vi "PH_Sound.ProcPeriodic.vi"(0 "i ref in":refnum<vi>, 3 "ms timeout (100)":i32=100, 5 "error in (no error)":errorcluster) -> (14 "i ref out":refnum<vi>, 17 "timed out":bool, 19 "error out":errorcluster)   [LabVIEW 2014, in "PH_Sound.lvlib"]
doc: "This method serves to periodically do things like reading values from the HW. Methods that should be executed periodically should be called from THIS methode. Add code here."
uses:
  PH_Sound.lvlib
  PH_Sound.3Oktaves.ctl
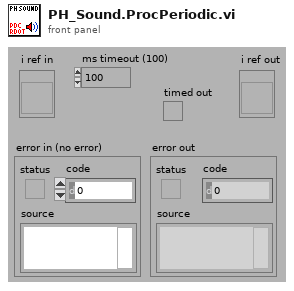
[diagram p1: front panel]
types:
  T1 = typedef "PH_Sound.lvlib/PH_Sound.i attribute.ctl" = cluster{"GUI Refs":cluster{"Exit":refnum<vi>, "Laserfreigabe":refnum<vi>, "PreAmp-Freigabe":refnum<vi>, "Countdown Running":refnum<vi>, "Emergency Off":refnum<vi>, "Device Error":refnum<vi>}, "Testalarm on":bool, "State":cluster{"Laser Class 4":bool, "PreAmp Running":bool, "Countdown Running":bool, "Emergency Off":bool}, "Starting Time":timestamp}
  T2 = typedef "PH_Sound.lvlib/PH_Sound.3Oktaves.ctl" = dbl
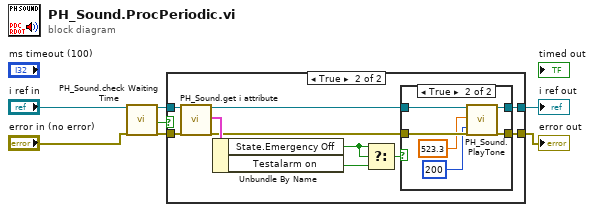
[diagram p0: block diagram]
diagram:
  n1 = call "PH_Sound.check Waiting Time.vi"("i ref in"="i ref in", "error in"="error in (no error)") -> ("i ref out"=w2:refnum<vi>, "Waiting Time over?"=w1:bool, "error out"=w4:errorcluster)  [unwired: 15 in]
  n2 = case shown="True" w1 {
    tunnel: [w9 w10] -> w7
    tunnel: [w8 w17] -> w6
    tunnel: w4 -> [w8 w12]
    tunnel: w2 -> [w9 w13]
    frame False {
    }
    frame True {
      n3 = call "PH_Sound.get i attribute.vi"("i ref in"=w13, "error in (no error)"=w12) -> ("i ref out"=w11:refnum<vi>, "i attribute"=w19:T1, "error out"=w18:errorcluster)  [unwired: 15 in]
      n4 = Unbundle By Name(w19) -> ("State.Emergency Off"=w16:bool, "Testalarm on"=w14:bool)
      n5 = Select(t=w16, s=w16, f=w14) -> (s? t:f=w15:bool)
      n6 = case shown="True" w15 {
        tunnel: w18 -> [w21 w27]
        tunnel: [w21 w26] -> w17
        tunnel: w11 -> [w20 w23]
        tunnel: [w20 w22] -> w10
        frame False {
        }
        frame True {
          w25 = T2 523.3 items=["c"=130.8, "cis"=138.6, "d"=146.8, "es"=155.6, "e"=164.8, "f"=174.6, "fis"=185.0, "g"=196.0, "as"=207.6, "a"=220.0, "b"=233.1, "h"=246.9, "c'"=261.6, "cis'"=277.2, "d'"=293.7, "es'"=311.1, "e'"=329.6, "f'"=349.2, "fis'"=370.0, "g'"=392.0, "as'"=415.3, "a'"=440.0, "b'"=466.2, "h'"=493.9, "c''"=523.3, "cis''"=554.4, "d''"=587.3, "es''"=622.3, "e''"=659.3, "f''"=689.5, "fis''"=740.0, "g''"=784.0, "as''"=830.6, "a''"=880.0, "b''"=932.3, "h''"=987.8, "c'''"=1047.0] ("tone")
          n7 = call "PH_Sound.PlayTone.vi"("VI in"=w23, "tone"=w25, "length [ms]"=200, "error in"=w27) -> ("VI out"=w22:refnum<vi>, "error out"=w26:errorcluster)  [unwired: 14 in]
        }
      }
    }
  }
  "error out" <- w6
  "i ref out" <- w7
